vi "test Initial Channel Values.vi"(8 "error in (no error)":errorcluster, 11 "TestCase in":refnum<class "Embedded Data Logger System Tests.lvclass">) -> (0 "error out":errorcluster, 3 "TestCase out":refnum<class "Embedded Data Logger System Tests.lvclass">)   [LabVIEW 2018, in "Embedded Data Logger System Tests.lvclass"]
uses:
  Embedded Data Logger System Tests.lvclass
  C:/Dev/niveristand-custom-device-testing-tools/VeriStandTestCase/VeriStandTestCase.lvclass
  <vilib>/NI Veristand/Execution/Workspace/NI VeriStand - Get Single Channel Value.vi
  <vilib>/addons/_JKI Toolkits/VI Tester/TestCase.llb/TestCase.lvclass
  <vilib>/NI Veristand/Execution/Workspace/NI_VS Workspace ExecutionAPI.lvlib
  C:/Program Files (x86)/National Instruments/LabVIEW 2018/vi.lib/addons/_JKI Toolkits/VI Tester/TestCase.llb/TestCase.lvclass
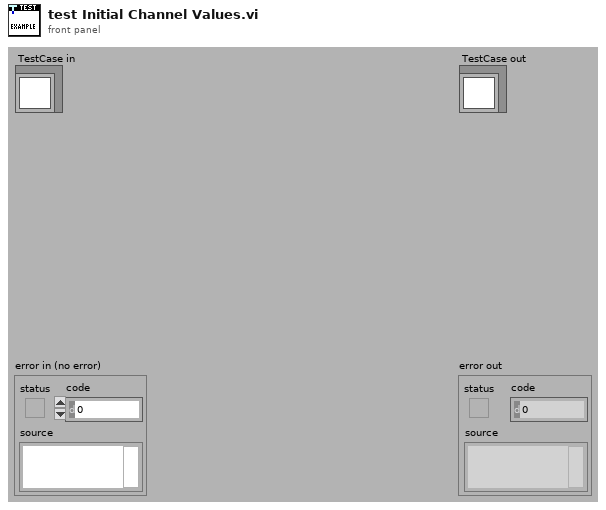
[diagram p1: front panel]
types:
  T1 = typedef "NI_VS Workspace ExecutionAPI.lvlib/WorkspaceAPI.ctl" = refnum<k24>
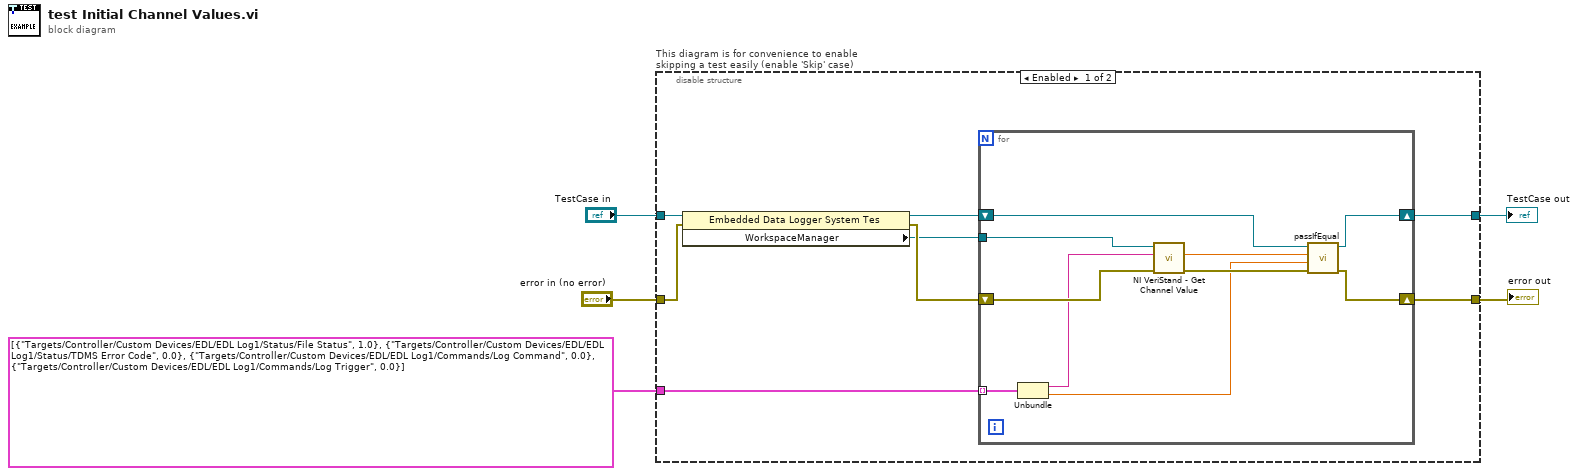
[diagram p0: block diagram]
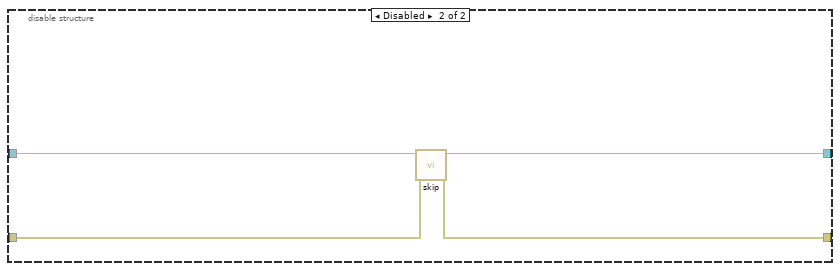
[diagram p2: hidden frame]
diagram:
  n1 = disable-structure "This diagram is for convenience to enable skipping a test easily (enable 'Skip' case)" shown="Enabled" {
    disable-tunnel: "TestCase in" -> [w11 w27]
    disable-tunnel: [w13 w25] -> w2
    disable-tunnel: [w12 w26] -> w4
    disable-tunnel: "error in (no error)" -> [w9 w24]
    disable-tunnel: cluster{string, dbl}[] [{"Targets/Controller/Custom Devices/EDL/EDL Log1/Status/File Status", 1.0}, {"Targets/Controller/Custom Devices/EDL/EDL Log1/Status/TDMS Error Code", 0.0}, {"Targets/Controller/Custom Devices/EDL/EDL Log1/Commands/Log Command", 0.0}, {"Targets/Controller/Custom Devices/EDL/EDL Log1/Commands/Log Trigger", 0.0}] -> [w6 _]
    frame Enabled {
      n2 = property class="Embedded Data Logger System Tes"(reference=w11, error in=w9) -> (reference out=w10:refnum<class "Embedded Data Logger System Tests.lvclass">, error out=w8:errorcluster, "WorkspaceManager"=w7:T1)
      n3 = for {
        tunnel: w7 -> [w18]
        shift-right: [w23] -> w13
        shift-left: w10 -> [w21]
        shift-right: [w22] -> w12
        shift-left: w8 -> [w20]
        tunnel: w6 -> [w17] mode=indexing
        n4 = Unbundle(w17) -> (w16:string, w15:dbl)
        n5 = call-poly <vilib>:"NI VeriStand - Get Channel Value.vi"("error in (no error)"=w20, "Channel"=w16, "WorkspaceManager in"=w18) -> ("error out"=w19:errorcluster, "Value"=w14:dbl)  [unwired: 6 in, 1 out]
        n6 = call-dynamic "passIfEqual.vi"("error in (no error)"=w19, "y"=w15, "x"=w14, "TestCase in"=w21) -> ("error out"=w22:errorcluster, "TestCase out"=w23:refnum<class "Embedded Data Logger System Tests.lvclass">)  [unwired: 6 in]
      }
    }
    frame Disabled {
      # "skip test result while test is under development"
      n7 = call <vilib>:"skip.vi"("error in (no error)"=w24, "TestCase in"=w27) -> ("error out"=w26:errorcluster, "TestCase out"=w25:refnum<class "Embedded Data Logger System Tests.lvclass">)  [unwired: 8 in]
    }
  }
  "error out" <- w4
  "TestCase out" <- w2
